vi "USBImageContinuousV1.4.vi"() -> ()   [LabVIEW 2019]
uses:
  C:/Users/Spenser Burrows/Desktop/Work/Labview software for spectrometer/PiezoStage_John/Piezojena.Protocols.Nv40Single.dll
  PiezoStage_John/Piezojena.Protocols.Nv40Single.dll
  <vilib>/Utility/file.llb/Write Delimited Spreadsheet (I64).vi
  Program Files (x86)/National Instruments/LabVIEW 2019/ATMCD32D.dll
  E:/PiezoStage_John/piezojena NV40Single.lvlib
panel:
  in  "Tab Control":T1(tab)
  out "Expected position on spectrometer (pixels):":dbl
  in  "Harmonic":dbl min=10.0 max=40.0
  out "l (nm)":dbl
  out "E (J)":dbl
  out "E (eV)":dbl
  out "Nearest Harmonic of 800nm":dbl
  out "Cursor Position (pixels)":dbl
  out "Distance to nearest harmonic of 800nm (pixels)":dbl
  in  "Grating:":u16(ring) items=["Shimadzu 30-006  "]
  in  "Laser:":u16(ring) items=["800nm  "]
  in  "Trigger":u32(ring) items=["Internal", "External"]
  out "Initialize":u32
  in  "Exposure Time (secs)":sgl format="%.2f"
  out "Calculated Exposure Value":sgl format="%.5f"
  out "Get Acquired Data":u32
  out "Start Acquisition":u32
  out "Detector X Pixels":i32
  out "Check Timings":u32
  out "Set Acquisition Mode":u32
  out "Set Readout Mode":u32
  out "Set Trigger Mode":u32
  out "Set Exposure Time":u32
  out "Get Detector":u32
  out "Detector Y Pixels":i32
  out "Shut Down":u32
  out "Set Gate Mode":u32
  out "Set Image":u32
  out "Raw Image From Camera":i32[][](graph)
  out "Vertical Binned Waveform Graph":i32[](graph)
  out "Get Status":u32
  in  "Stop":bool
  in  "Save image":bool
  out "Camera Status:":bool
  out "Last Image Saved:":string
  out "Wavelength Graph (nm)":cluster{"No prefix":dbl, i32}[](graph)
  out "Energy Graph (eV)":cluster{"eV":dbl, i32}[](graph)
  out "Harmonics Graph":cluster{"No prefix":dbl, i32}[](graph)
  in  "Measurement Length [fs]":ext=30.0
  out "Optical Cycles \nin measurement":ext=16.905589736842103296
  in  "Initial Piezo Position":sgl=40.0
  out "Number of Steps":ext=300.00000000000005795
  in  "Step Size [as]":sgl=100.0
  in  "?":bool
  in  "Settings":bool
  in  "Wavelength (nm)":i32(listbox)
  in  "Piezojena Seriel Port":refnum<visa-resource-name>="COM4"
  out "Piezo Voltage Supply":cluster{dbl[], dbl[]}(graph)={[0.0], [70.08999633789062]}
  in  "Initial Piezo Position [um]":dbl(slide)=40.0 scale=0.0..80.0
  in  "Final Piezo Position [um]":dbl(slide)=48.99377374 scale=0.0..80.0
  out "Volt Meter":dbl(knob)=70.08999633789062 scale=-10.0..150.0
  out "Raw Image From Camera":i32[][](graph)
  out "Status":u32
  # "Status"
  # "Return values"
  # "Acquisition Mode: Single Scan\nReadout Mode: Full Resolution Image"
  # "XUV Spectrometer Control VI"
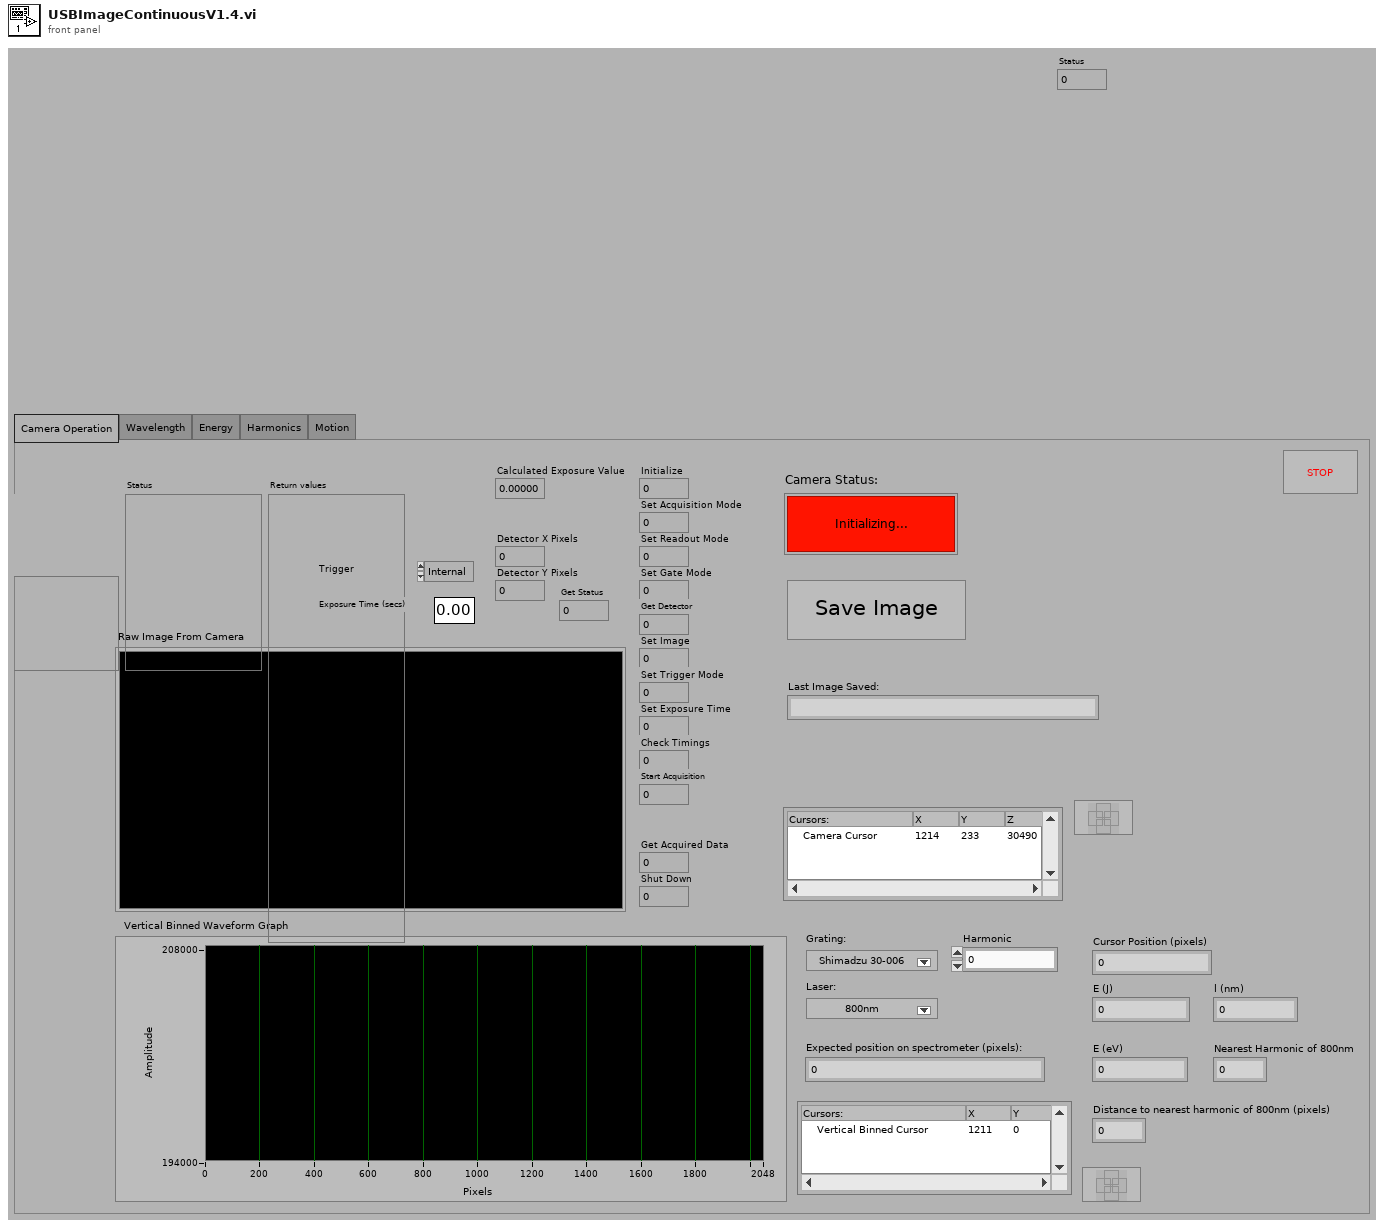
[diagram p1: front panel]
types:
  T1 = enum32{"Camera Operation", "Wavelength", "Energy", "Harmonics", "Motion"}
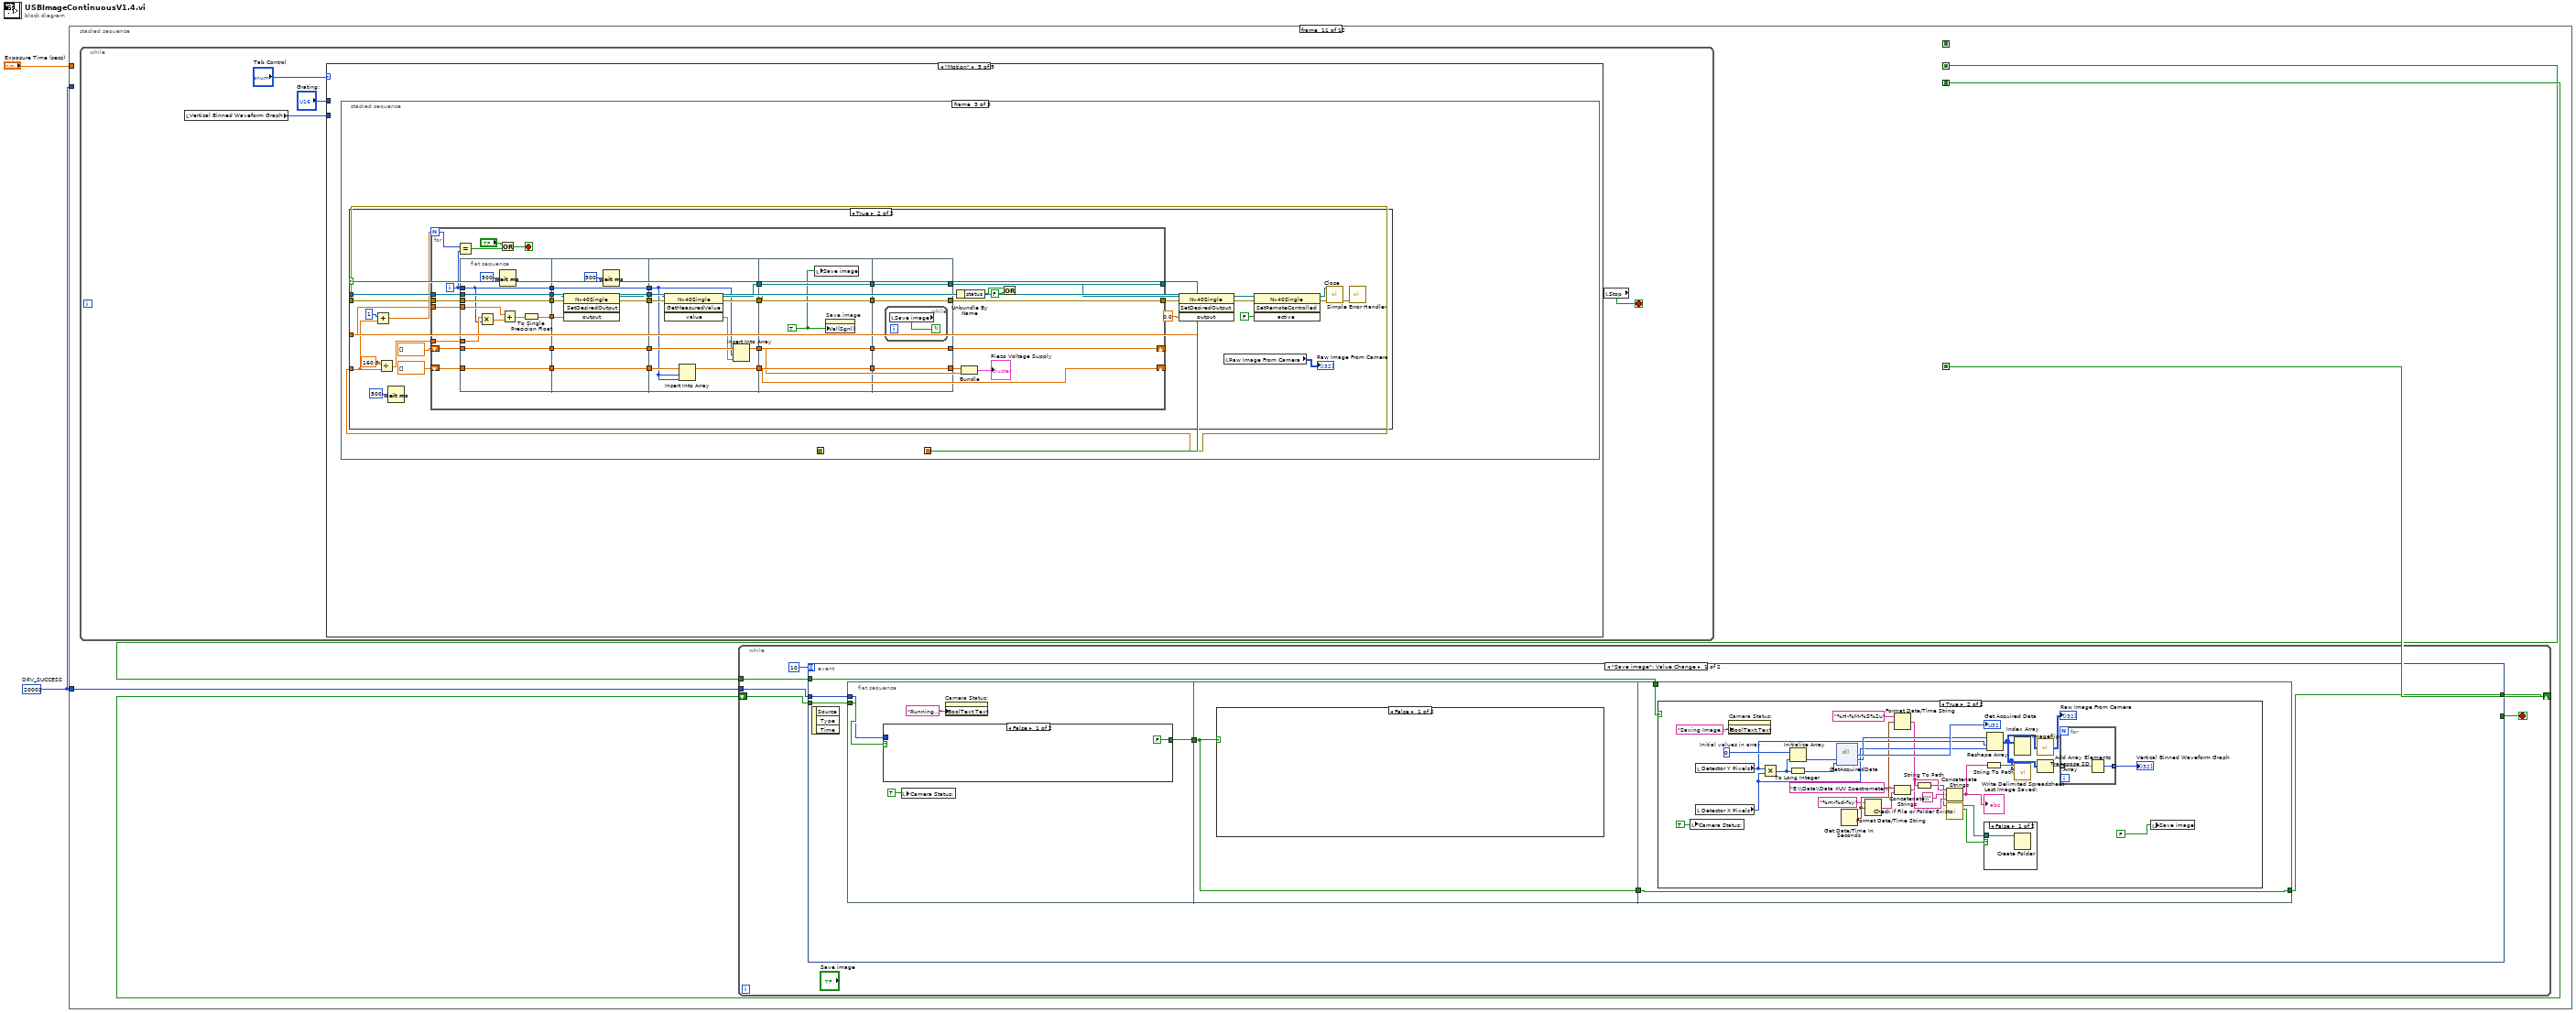
[diagram p0: block diagram]
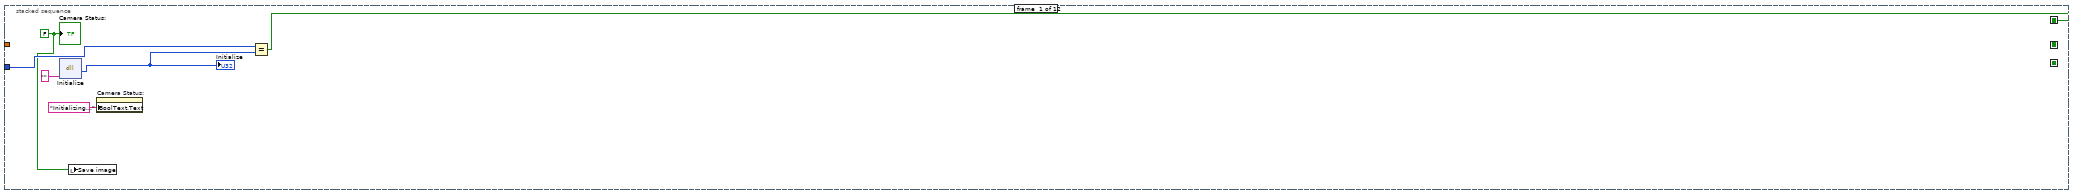
[diagram p2: hidden frame]
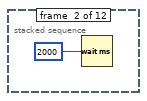
[diagram p3: hidden frame]
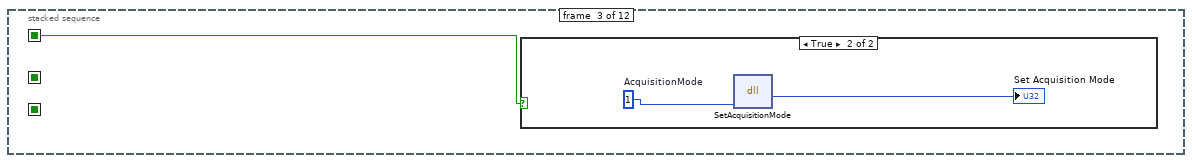
[diagram p4: hidden frame]
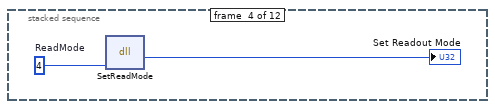
[diagram p6: hidden frame]
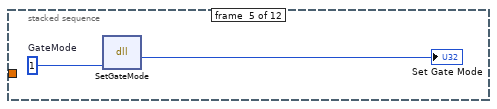
[diagram p7: hidden frame]
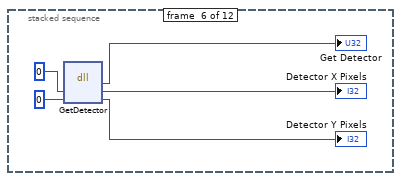
[diagram p8: hidden frame]
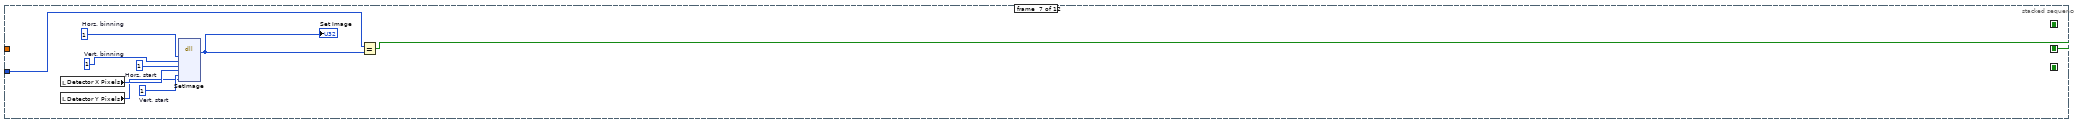
[diagram p9: hidden frame]
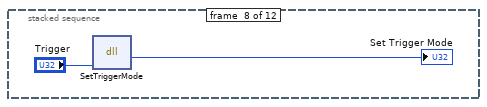
[diagram p10: hidden frame]
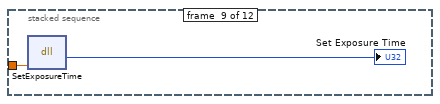
[diagram p11: hidden frame]
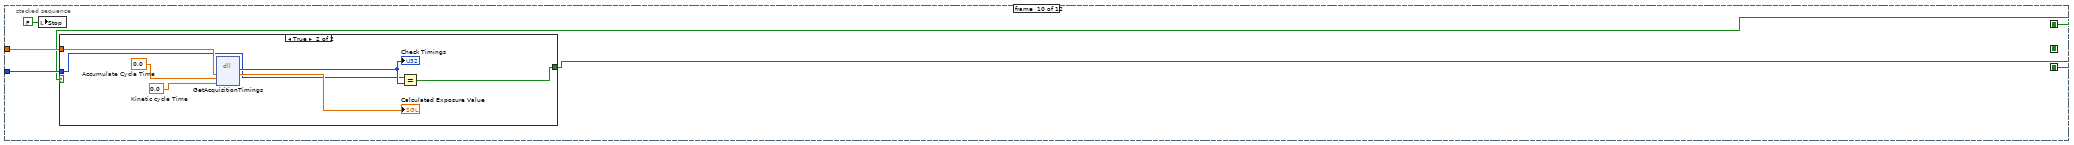
[diagram p12: hidden frame]
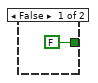
[diagram p13: hidden frame]
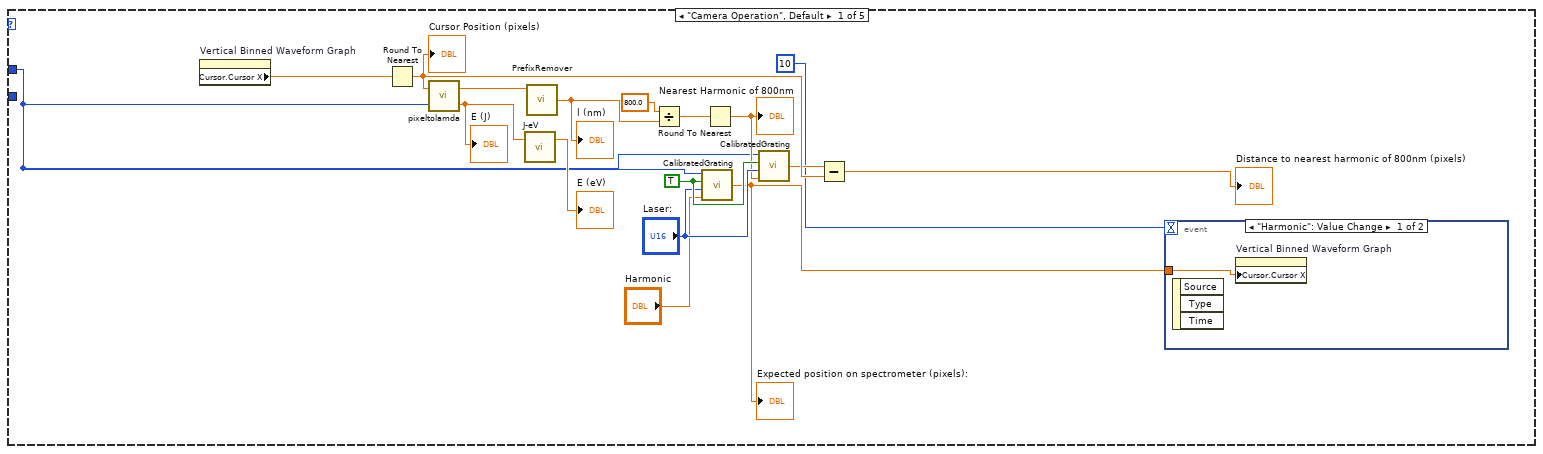
[diagram p14: hidden frame]
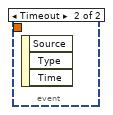
[diagram p15: hidden frame]
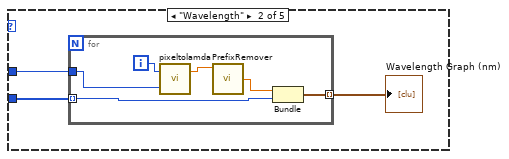
[diagram p16: hidden frame]
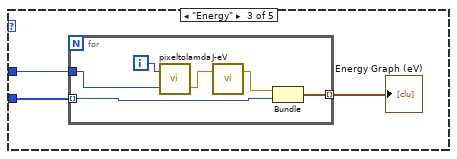
[diagram p17: hidden frame]
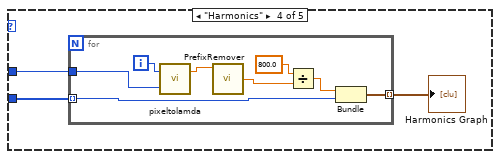
[diagram p18: hidden frame]
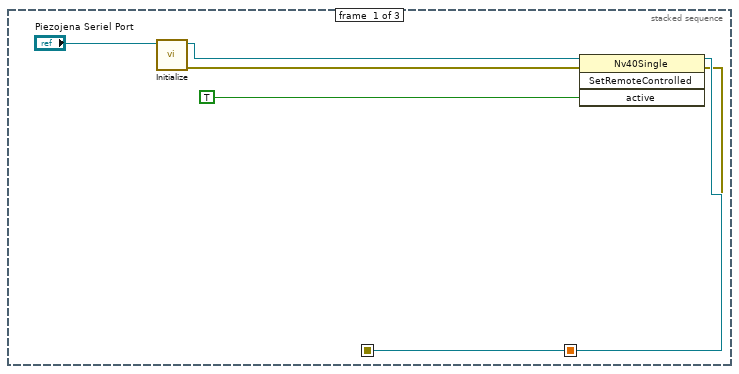
[diagram p19: hidden frame]
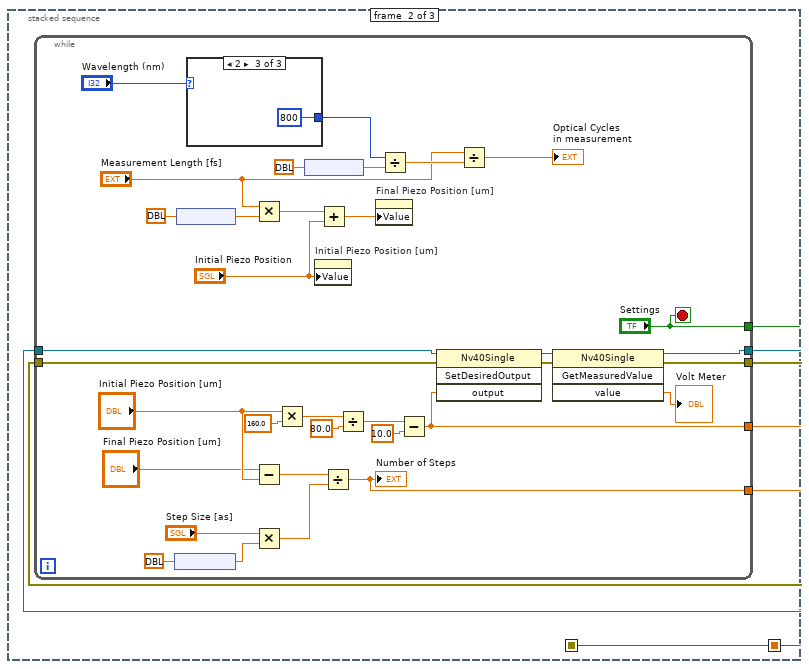
[diagram p20: hidden frame]
diagram:
  w1 = 20002  # DRV_SUCCESS
  n1 = stacked-sequence {
    seq-local: [w6 _ _ _ _ _ _ _ _ _ _ _] -> [_ _ w10 _ _ _ _ _ _ w36 _ w370]
    seq-local: [_ _ _ _ _ _ _ _ _ w37 _ _] -> [_ _ _ _ _ _ _ _ _ _ w51 _]
    seq-local: [_ _ _ _ _ _ _ _ _ _ w49 _] -> [_ _ _ _ _ _ _ _ _ _ _ _]
    seq-local: [_ _ _ _ _ _ w22 _ _ _ _ _] -> [_ _ _ _ _ _ _ _ _ _ w48 _]
    tunnel: "Exposure Time (secs)" -> [_ _ _ _ _ _ _ _ w34 w39 _ _]
    tunnel: w1 -> [w7 _ _ _ _ _ w24 _ _ w38 _ _]
    tunnel: w1 -> [_ _ _ _ _ _ _ _ _ _ w50 _]
    frame #0 {
      w3 = FALSE ("Camera Status:")
      n2 = dll-call lib="C:/Program Files (x86)/National Instruments/LabVIEW 2019/atmcd32d.dll" fn="Initialize" label="Call Library Function Initialize"("") -> (w8:u32)  [unwired: 4 in, 2 out]
      "Initialize" <- w8
      n3 = local write "Save image"(w3) -> ()
      n4 = property on="Camera Status:" class="Bool (strict)"("BoolText.Text"="Initializing..." ("String")) -> ()  [unwired: 2 in, 2 out]
      n5 = Equal?(x=w7, y=w8) -> (x = y?=w6:bool)
      "Camera Status:" <- w3
    }
    frame #1 {
      n6 = Wait (ms)(milliseconds to wait=u32 2000) -> ()  [unwired: 1 out]
    }
    frame #2 {
      n7 = case shown="True" w10 {
        frame False {
        }
        frame True {
          w12 = u16 1  # AcquisitionMode
          n8 = dll-call lib="C:/Program Files (x86)/National Instruments/LabVIEW 2019/atmcd32d.dll" fn="SetAcquisitionMode" label="Call Library Function SetAcquisitionMode"(w12) -> (→"Set Acquisition Mode":u32)  [unwired: 4 in, 2 out]
        }
      }
    }
    frame #3 {
      w14 = u16 4  # ReadMode
      n9 = dll-call lib="C:/Program Files (x86)/National Instruments/LabVIEW 2019/atmcd32d.dll" fn="SetReadMode" label="Call Library Function SetReadMode"(w14) -> (→"Set Readout Mode":u32)  [unwired: 4 in, 2 out]
    }
    frame #4 {
      w16 = u16 1  # GateMode
      n10 = dll-call lib="C:/Program Files (x86)/National Instruments/LabVIEW 2019/atmcd32d.dll" fn="SetGateMode" label="Call Library Function SetGateMode"(w16) -> (→"Set Gate Mode":u32)  [unwired: 4 in, 2 out]
    }
    frame #5 {
      n11 = dll-call lib="C:/Program Files (x86)/National Instruments/LabVIEW 2019/atmcd32d.dll" fn="GetDetector" label="Call Library FunctionGetDetector"(i16 0, i16 0) -> (→"Get Detector":u32, →"Detector X Pixels":i32, →"Detector Y Pixels":i32)  [unwired: 3 in, 2 out]
    }
    frame #6 {
      w27 = u16 1  # Vert. start
      w28 = u16 1  # Horz. start
      w29 = u16 1  # Vert. binning
      w30 = u16 1  # Horz. binning
      n12 = local read "Detector X Pixels"() -> (w26:i32)
      n13 = local read "Detector Y Pixels"() -> (w25:i32)
      n14 = dll-call lib="C:/Program Files (x86)/National Instruments/LabVIEW 2019/atmcd32d.dll" fn="SetImage" label="Call Library Function SetImage"(w30, w29, w28, w26, w27, w25) -> (w23:u32)  [unwired: 9 in, 2 out]
      "Set Image" <- w23
      n15 = Equal?(x=w24, y=w23) -> (x = y?=w22:bool)
    }
    frame #7 {
      n16 = dll-call lib="C:/Program Files (x86)/National Instruments/LabVIEW 2019/atmcd32d.dll" fn="SetTriggerMode" label="Call Library Function SetTrigger Mode"("Trigger") -> (→"Set Trigger Mode":u32)  [unwired: 4 in, 2 out]
    }
    frame #8 {
      n17 = dll-call lib="C:/Program Files (x86)/National Instruments/LabVIEW 2019/atmcd32d.dll" fn="SetExposureTime" label="Call Library FunctionSet Exposure Time"(w34) -> (→"Set Exposure Time":u32)  [unwired: 4 in, 2 out]
    }
    frame #9 {
      n18 = local write "Stop"(FALSE ("Stop")) -> ()
      n19 = case shown="True" w36 {
        tunnel: w39 -> [_ w44]
        tunnel: w38 -> [_ w41]
        tunnel: [FALSE w43] -> w37
        frame False {
        }
        frame True {
          w46 = sgl 0.0  # Accumulate Cycle Time
          w47 = sgl 0.0  # Kinetic cycle Time
          n20 = dll-call lib="C:/Program Files (x86)/National Instruments/LabVIEW 2019/atmcd32d.dll" fn="GetAcquisitionTimings" label="Call Library Function Check Timings"(w44, w46, w47) -> (w42:u32, →"Calculated Exposure Value":sgl)  [unwired: 5 in, 2 out]
          "Check Timings" <- w42
          n21 = Equal?(x=w41, y=w42) -> (x = y?=w43:bool)
        }
      }
    }
    frame #10 {
      n22 = while {
        stop <- w52 stop-if-true
        n23 = local read "Vertical Binned Waveform Graph"() -> (w54:i32[])
        n24 = case shown="\"Motion\"" "Tab Control" {
          tunnel: w54 -> [_ w76 w85 w94 _]
          tunnel: "Grating:" -> [w56 w75 w84 w93 _]
          frame "Camera Operation", Default {
            w72 = TRUE
            n25 = property on="Vertical Binned Waveform Graph" class="WFGraph (strict)"() -> ("Cursor.Cursor X"=w69:dbl)  [unwired: 2 in, 2 out]
            n26 = Round To Nearest(number=w69) -> (nearest integer value=w62:dbl)
            "Cursor Position (pixels)" <- w62
            n27 = call "pixeltolamda.vi"("Grating:"=w56, "Pixel Postion"=w62) -> ("E (J)"=w64:dbl, "lamda (m)"=w70:dbl)
            "E (J)" <- w64
            n28 = call "J-eV.vi"("J"=w64) -> ("eV"=→"E (eV)":dbl)  [unwired: 1 in, 1 out]
            n29 = call "PrefixRemover.vi"("Nano"=w70) -> ("No prefix"=w65:dbl)  [unwired: 3 in]
            "l (nm)" <- w65
            n30 = Divide(x=800.0, y=w65) -> (x/y=w67:dbl)
            n31 = call "CalibratedGrating.vi"("Harmonic"="Harmonic", "Laser:"="Laser:", "Subvi?"=w72, "Grating:"=w56) -> ("Position on spectrometer (pixels):"=w58:dbl)
            "Expected position on spectrometer (pixels):" <- w58
            n32 = Round To Nearest(number=w67) -> (nearest integer value=w61:dbl)
            "Nearest Harmonic of 800nm" <- w61
            n33 = call "CalibratedGrating.vi"("Harmonic"=w61, "Laser:"="Laser:", "Subvi?"=w72, "Grating:"=w56) -> ("Position on spectrometer (pixels):"=w60:dbl)
            n34 = Subtract(x=w60, y=w62) -> (x-y=→"Distance to nearest harmonic of 800nm (pixels)":dbl)
            n35 = event shown="[0] \"Harmonic\": Value Change" {
              selector: _ -> [_ _]
              dyn-events: _ -> [_ _]
              timeout: 10 -> [_ _]
              tunnel: w58 -> [w73 _]
              event "Harmonic": Value Change {
                n36 = event-data() -> ()  [unwired: 1 in, 3 out]
                n37 = property on="Vertical Binned Waveform Graph" class="WFGraph (strict)"("Cursor.Cursor X"=w73) -> ()  [unwired: 2 in, 2 out]
              }
              event Timeout {
                n38 = event-data() -> ()  [unwired: 1 in, 3 out]
              }
            }
          }
          frame "Wavelength" {
            n39 = for {
              tunnel: w76 -> [w78] mode=indexing
              tunnel: w75 -> [w80]
              tunnel: [w77] -> w74 mode=indexing
              i -> [w79]
              n40 = call "pixeltolamda.vi"("Grating:"=w80, "Pixel Postion"=w79) -> ("lamda (m)"=w81:dbl)  [unwired: 1 out]
              n41 = call "PrefixRemover.vi"("Nano"=w81) -> ("No prefix"=w82:dbl)  [unwired: 3 in]
              n42 = Bundle("No prefix"=w82, w78) -> (w77:cluster{"No prefix":dbl, i32})  [unwired: 1 in]
            }
            "Wavelength Graph (nm)" <- w74
          }
          frame "Energy" {
            n43 = for {
              tunnel: w85 -> [w87] mode=indexing
              tunnel: w84 -> [w90]
              tunnel: [w86] -> w83 mode=indexing
              i -> [w91]
              n44 = call "pixeltolamda.vi"("Grating:"=w90, "Pixel Postion"=w91) -> ("E (J)"=w89:dbl)  [unwired: 1 out]
              n45 = call "J-eV.vi"("J"=w89) -> ("eV"=w88:dbl)  [unwired: 1 in, 1 out]
              n46 = Bundle("eV"=w88, w87) -> (w86:cluster{"eV":dbl, i32})  [unwired: 1 in]
            }
            "Energy Graph (eV)" <- w83
          }
          frame "Harmonics" {
            n47 = for {
              tunnel: w94 -> [w99] mode=indexing
              tunnel: w93 -> [w101]
              tunnel: [w98] -> w92 mode=indexing
              i -> [w100]
              n48 = call "pixeltolamda.vi"("Grating:"=w101, "Pixel Postion"=w100) -> ("lamda (m)"=w102:dbl)  [unwired: 1 out]
              n49 = call "PrefixRemover.vi"("Nano"=w102) -> ("No prefix"=w96:dbl)  [unwired: 3 in]
              n50 = Divide(x=800.0, y=w96) -> (x/y=w95:dbl)
              n51 = Bundle(w95, w99) -> (w98:cluster{dbl, i32})  [unwired: 1 in]
            }
            "Harmonics Graph" <- w92
          }
          frame "Motion" {
            n52 = stacked-sequence {
              seq-local: [w104 _ _] -> [_ w115 _]
              seq-local: [w103 _ _] -> [_ w114 _]
              seq-local: [_ w113 _] -> [_ _ w157]
              seq-local: [_ w112 _] -> [_ _ w156]
              seq-local: [_ w111 _] -> [_ _ w155]
              seq-local: [_ w110 _] -> [_ _ w154]
              seq-local: [_ w109 _] -> [_ _ w153]
              frame #0 {
                n53 = call "Initialize.vi"("VISA resource name"="Piezojena Seriel Port") -> ("error out"=w108:errorcluster, "Piezojena.Protocols.Nv40Single.Nv40Single"=w107:refnum<k24>)  [unwired: 9 in]
                n54 = invoke class="Nv40Single" method="SetRemoteControlled"(reference=w107, error in=w108, "active"=TRUE) -> (reference out=w104:refnum<k24>, error out=w103:errorcluster)  [unwired: 1 in, 2 out]
              }
              frame #1 {
                n55 = while {
                  tunnel: ["Settings"] -> w113
                  tunnel: [w136] -> w112
                  tunnel: [w148] -> w111
                  tunnel: [w147] -> w110
                  tunnel: w115 -> [w146]
                  tunnel: w114 -> [w145]
                  tunnel: [w130] -> w109
                  stop <- "Settings" stop-if-true
                  n56 = node(ext[unit] 299792458.0) -> (w134:ext)
                  n57 = node(ext[unit] 299792458.0) -> (w121:ext)
                  n58 = case shown="2" "Wavelength (nm)" {
                    tunnel: [532 ("Numeric 2") 633 ("Numeric 2") 800 ("Numeric 2")] -> w125
                    frame 0, Default {
                    }
                    frame 1 {
                    }
                    frame 2 {
                    }
                  }
                  n59 = Multiply(x="Measurement Length [fs]", y=w121) -> (x*y=w119:ext)
                  n60 = Subtract(x="Final Piezo Position [um]", y="Initial Piezo Position [um]") -> (x-y=w133:dbl)
                  n61 = Multiply(x="Step Size [as]", y=w134) -> (x*y=w132:ext)
                  n62 = Multiply(x="Initial Piezo Position [um]", y=160.0 ("x")) -> (x*y=w139:dbl)
                  n63 = node(ext[unit] 299792458.0) -> (w124:ext)
                  n64 = property on="Initial Piezo Position [um]" class="Slide (strict)"("Value"="Initial Piezo Position") -> ()  [unwired: 2 in, 2 out]
                  n65 = Add(x=w119, y="Initial Piezo Position") -> (x+y=w118:ext)
                  n66 = Divide(x=w133, y=w132) -> (x/y=w130:ext)
                  "Number of Steps" <- w130
                  n67 = Divide(x=w139, y=80.0) -> (x/y=w138:dbl)
                  n68 = property on="Final Piezo Position [um]" class="Slide (strict)"("Value"=w118) -> ()  [unwired: 2 in, 2 out]
                  n69 = Divide(x=w125, y=w124) -> (x/y=w117:ext)
                  n70 = Subtract(x=w138, y=10.0) -> (x-y=w136:dbl)
                  n71 = invoke class="Nv40Single" method="SetDesiredOutput"(reference=w146, error in=w145, "output"=w136) -> (reference out=w142:refnum<k24>, error out=w143:errorcluster)  [unwired: 1 in, 2 out]
                  n72 = Divide(x="Measurement Length [fs]", y=w117) -> (x/y=→"Optical Cycles \nin measurement":ext)
                  n73 = invoke class="Nv40Single" method="GetMeasuredValue"(reference=w142, error in=w143) -> (reference out=w148:refnum<k24>, error out=w147:errorcluster, "value"=→"Volt Meter":sgl)  [unwired: 2 in, 1 out]
                }
              }
              frame #2 {
                n74 = case shown="True" w157 {
                  tunnel: w156 -> [_ w171]
                  tunnel: w155 -> [_ w170]
                  tunnel: w154 -> [_ w169]
                  tunnel: w153 -> [_ w165]
                  frame False {
                    (unwired) TRUE ("Stop Measurement 2")
                  }
                  frame True {
                    n75 = Add(x=1 ("y"), y=w165) -> (x+y=w172:ext)
                    n76 = Divide(x=160.0, y=w165) -> (x/y=w164:ext)
                    n77 = Wait (ms)(milliseconds to wait=u32 500 ("Wait for \nPiezo to start 2")) -> ()  [unwired: 1 out]
                    n78 = for {
                      N: w172 -> [w213]
                      tunnel: [w215] -> w163
                      tunnel: [w214] -> w162
                      tunnel: w170 -> [w205]
                      tunnel: w169 -> [w204]
                      tunnel: w171 -> [w200]
                      shift-right: [w188] -> _
                      shift-left: dbl[] [] -> [w198]
                      shift-right: [w189] -> _
                      shift-left: dbl[] [] -> [w193]
                      tunnel: w164 -> [w187]
                      i -> [w199]
                      stop <- w212 stop-if-true
                      n79 = Equal?(x=w213, y=w199) -> (x = y?=w211:bool)
                      n80 = flat-sequence {
                        tunnel: w204 -> [w225]
                        tunnel: w205 -> [w226]
                        tunnel: [w226] -> w203
                        tunnel: [w225] -> w202
                        tunnel: [w221] -> w201
                        tunnel: w199 -> [w218]
                        tunnel: w187 -> [w223]
                        tunnel: w200 -> [w222]
                        tunnel: w198 -> [w219]
                        tunnel: [w219] -> w197
                        tunnel: [w218] -> w194
                        tunnel: w193 -> [w216]
                        tunnel: [w216] -> w192
                        tunnel: [w231] -> w209
                        tunnel: [w230] -> w208
                        tunnel: w203 -> [w234]
                        tunnel: w202 -> [w233]
                        tunnel: w201 -> [w232]
                        tunnel: w197 -> [w229]
                        tunnel: [w229] -> w196
                        tunnel: [w228] -> w195
                        tunnel: w194 -> [w228]
                        tunnel: w192 -> [w227]
                        tunnel: [w227] -> w191
                        tunnel: w209 -> [w242]
                        tunnel: w208 -> [w241]
                        tunnel: w196 -> [w240]
                        tunnel: w195 -> [w237]
                        tunnel: w191 -> [w238]
                        tunnel: [w245] -> w186
                        tunnel: [w244] -> w185
                        tunnel: [w243] -> w184
                        tunnel: [w239] -> w183
                        tunnel: w186 -> [w250]
                        tunnel: w185 -> [w249]
                        tunnel: w184 -> [w248]
                        tunnel: w183 -> [w247]
                        tunnel: [w250] -> w182
                        tunnel: [w249] -> w181
                        tunnel: [w248] -> w180
                        tunnel: [w247] -> w179
                        tunnel: [w251] -> w189
                        tunnel: [w252] -> w188
                        tunnel: [w253] -> w214
                        tunnel: [w254] -> w215
                        tunnel: w182 -> [w254]
                        tunnel: w181 -> [w253]
                        tunnel: w180 -> [w252]
                        tunnel: w179 -> [w251]
                        frame #0 {
                          n81 = Multiply(x=w223, y=w218) -> (x*y=w217:ext)
                          n82 = Wait (ms)(milliseconds to wait=u32 500 ("Delay (ms) 3")) -> ()  [unwired: 1 out]
                          n83 = Add(x=w222, y=w217) -> (x+y=w224:ext)
                          n84 = To Single Precision Float(number=w224) -> (single precision float=w221:sgl)
                        }
                        frame #1 {
                          n85 = invoke class="Nv40Single" method="SetDesiredOutput"(reference=w234, error in=w233, "output"=w232) -> (reference out=w231:refnum<k24>, error out=w230:errorcluster)  [unwired: 1 in, 2 out]
                          n86 = Wait (ms)(milliseconds to wait=u32 500 ("Delay (ms) 4")) -> ()  [unwired: 1 out]
                        }
                        frame #2 {
                          n87 = invoke class="Nv40Single" method="GetMeasuredValue"(reference=w242, error in=w241) -> (reference out=w245:refnum<k24>, error out=w244:errorcluster, "value"=w236:sgl)  [unwired: 2 in, 1 out]
                          n88 = Insert Into Array(array=w238, index=w237, new element=w237) -> (w239:dbl[])
                          n89 = Insert Into Array(array=w240, index=w237, new element=w236) -> (w243:dbl[])
                        }
                        frame #3 {
                          w246 = TRUE
                          n90 = local write "Save image"(w246) -> ()
                          n91 = property on="Save image" class="Bool (strict)"("Val(Sgnl)"=w246) -> ()  [unwired: 2 in, 2 out]
                        }
                        frame #4 {
                          n92 = while {
                            stop <- w255 continue-if-true
                            n93 = local read "Save image"() -> (w255:bool)
                          }
                        }
                      }
                      n94 = Or(x="?", y=w211) -> (x .or. y?=w212:bool)
                      n95 = Unbundle By Name(w214) -> ("status"=w207:bool)
                      n96 = Bundle(w189, w188) -> (→"Piezo Voltage Supply":cluster{dbl[], dbl[]})  [unwired: 1 in]
                      n97 = Or(x=w207, y=FALSE ("Halt Measurment")) -> ()  [unwired: 1 out]
                    }
                    n98 = invoke class="Nv40Single" method="SetDesiredOutput"(reference=w163, error in=w162, "output"=sgl 0.0) -> (reference out=w160:refnum<k24>, error out=w159:errorcluster)  [unwired: 1 in, 2 out]
                    n99 = local read "Raw Image From Camera"() -> (→"Raw Image From Camera":i32[][])
                    n100 = invoke class="Nv40Single" method="SetRemoteControlled"(reference=w160, error in=w159, "active"=FALSE) -> (reference out=w177:refnum<k24>, error out=w175:errorcluster)  [unwired: 1 in, 2 out]
                    n101 = call "Close.vi"("error in (no error)"=w175, "reference"=w177) -> ("error out"=w178:errorcluster)  [unwired: 9 in]
                    n102 = call <vilib>:"Simple Error Handler.vi"("error in (no error)"=w178) -> ()  [unwired: 4 in, 5 out]
                  }
                }
              }
            }
          }
        }
        n103 = local read "Stop"() -> (w52:bool)
      }
      n104 = while {
        tunnel: w50 -> [w260]
        tunnel: w48 -> [w258]
        shift-right: [w259] -> w49
        shift-left: w51 -> [w261]
        stop <- w256 stop-if-true
        n105 = event shown="[0] \"Save image\": Value Change" {
          selector: _ -> [_ _]
          dyn-events: _ -> [_ _]
          timeout: 10 -> [_ _]
          tunnel: w261 -> [w265 w322]
          tunnel: w260 -> [w264 w321]
          tunnel: [w263 w320] -> w259
          tunnel: w258 -> [w262 w319]
          tunnel: [_ w318] -> w256
          event "Save image": Value Change {
            n106 = event-data() -> ()  [unwired: 1 in, 3 out]
            n107 = flat-sequence {
              tunnel: w265 -> [w272]
              tunnel: w264 -> [w271]
              tunnel: [w270] -> w267
              tunnel: w267 -> [w277]
              tunnel: [w277] -> w266
              tunnel: [w285] -> w263
              tunnel: w266 -> [w285]
              tunnel: w262 -> [w284]
              frame #0 {
                n108 = case shown="False" w272 {
                  tunnel: [FALSE w275] -> w270
                  tunnel: w271 -> [_ w274]
                  frame False {
                  }
                  frame True {
                    n109 = dll-call lib="C:/Program Files (x86)/National Instruments/LabVIEW 2019/atmcd32d.dll" fn="StartAcquisition" label="Call Library Function start acquisition"() -> (w276:u32)  [unwired: 3 in, 2 out]
                    "Start Acquisition" <- w276
                    n110 = Equal?(x=w274, y=w276) -> (x = y?=w275:bool)
                  }
                }
                n111 = local write "Camera Status:"(TRUE ("Camera Status:")) -> ()
                n112 = property on="Camera Status:" class="Bool (strict)"("BoolText.Text"="Running..." ("Boolean Text.Text")) -> ()  [unwired: 2 in, 2 out]
              }
              frame #1 {
                n113 = case shown="False" w277 {
                  frame False {
                  }
                  frame True {
                    n114 = while {
                      stop <- w281 continue-if-true
                      w280 = u16 20072  # DRV ACQUIRING
                      n115 = Wait Until Next ms Multiple(millisecond multiple=u32 500) -> ()  [unwired: 1 out]
                      n116 = dll-call lib="C:/Program Files (x86)/National Instruments/LabVIEW 2019/atmcd32d.dll" fn="GetStatus" label="Call Library Function GetAcquisitionStatus"(u16 0) -> (→"Get Status":u32, w279:u32)  [unwired: 3 in, 2 out]
                      "Status" <- w279
                      n117 = Equal?(x=w279, y=w280) -> (x = y?=w281:bool)
                    }
                  }
                }
              }
              frame #2 {
                n118 = case shown="True" w284 {
                  frame False {
                  }
                  frame True {
                    w313 = 0  # Initial values in array
                    n119 = local write "Camera Status:"(TRUE ("Camera Status:")) -> ()
                    n120 = local read "Detector Y Pixels"() -> (w307:i32)
                    n121 = local read "Detector X Pixels"() -> (w306:i32)
                    n122 = property on="Camera Status:" class="Bool (strict)"("BoolText.Text"="Saving Image..." ("Boolean Text.Text")) -> ()  [unwired: 2 in, 2 out]
                    n123 = Multiply(x=w307, y=w306) -> (x*y=w309:i32)
                    n124 = To Long Integer(number=w309) -> (32bit integer=w310:i32)
                    n125 = Initialize Array "Initialize Array"(w313, w309) -> (w311:i32[])
                    n126 = dll-call lib="C:/Program Files (x86)/National Instruments/LabVIEW 2019/atmcd32d.dll" fn="GetAcquiredData" label="Call Library Function Get Acquired data"(w311, w310) -> (→"Get Acquired Data":u32, w308:i32[])  [unwired: 4 in, 2 out]
                    n127 = Get Date/Time In Seconds() -> (seconds since 1Jan1904=w303:timestamp)
                    n128 = Format Date/Time String(time format string (%c)="%m-%d-%y", seconds (now)=w303) -> (date/time string=w301:string)  [unwired: 1 in]
                    n129 = Format Date/Time String(time format string (%c)="%H-%M-%S%2u", seconds (now)=w303) -> (date/time string=w302:string)  [unwired: 1 in]
                    n130 = Concatenate Strings("E:\\Data\\Data XUV Spectrometer\\" ("string"), w301) -> (w304:string)
                    n131 = String To Path(string=w304) -> (path=w300:path)
                    n132 = Concatenate Strings(w304, "\\" ("string"), w302) -> (w305:string)
                    "Last Image Saved:" <- w305
                    n133 = call <vilib>:"Check if File or Folder Exists.vi"("path"=w300) -> ("file or folder exists?"=w298:bool, "dup path"=w299:path)  [unwired: 8 in, 1 out]
                    n134 = case shown="False" w298 {
                      tunnel: w299 -> [w316 _]
                      frame False {
                        n135 = Create Folder(path (use dialog)=w316) -> ()  [unwired: 2 in, 3 out]
                      }
                      frame True {
                      }
                    }
                    n136 = String To Path(string=w305) -> (path=w293:path)
                    n137 = Reshape Array(w308, w307, w306) -> (w288:i32[][])
                    n138 = Index Array(array=w288) -> ()  [unwired: 2 in, 1 out]
                    n139 = call-poly <vilib>:"Write Delimited Spreadsheet.vi"("file path (dialog if empty)"=w293, "2D data"=w288) -> ()  [unwired: 12 in, 2 out]
                    n140 = call "Imageflip.vi"("2D array"=w288) -> ("transposed array"=→"Raw Image From Camera":i32[][])
                    n141 = Transpose 2D Array(2D array=w288) -> (transposed array=w292:i32[][])
                    n142 = for {
                      tunnel: w292 -> [w315] mode=indexing
                      tunnel: [w314] -> w291 mode=indexing
                      n143 = Add Array Elements(numeric array=w315) -> (sum=w314:i32)
                    }
                    "Vertical Binned Waveform Graph" <- w291
                    n144 = local write "Save image"(FALSE ("Take image")) -> ()
                  }
                }
              }
            }
          }
          event Timeout {
            n145 = event-data() -> ()  [unwired: 1 in, 3 out]
            n146 = flat-sequence {
              tunnel: w322 -> [w329]
              tunnel: w321 -> [w328]
              tunnel: [w327] -> w324
              tunnel: w324 -> [w334]
              tunnel: [w334] -> w323
              tunnel: w323 -> [w341]
              tunnel: w319 -> [w342]
              tunnel: [w341] -> w317
              tunnel: ["Stop"] -> w318
              tunnel: [w367] -> w320
              tunnel: w317 -> [w367]
              frame #0 {
                n147 = case shown="True" w329 {
                  tunnel: [FALSE w333] -> w327
                  tunnel: w328 -> [_ w332]
                  frame False {
                  }
                  frame True {
                    n148 = dll-call lib="C:/Program Files (x86)/National Instruments/LabVIEW 2019/atmcd32d.dll" fn="StartAcquisition" label="Call Library Function start acquisition"() -> (w331:u32)  [unwired: 3 in, 2 out]
                    n149 = local write "Start Acquisition"(w331) -> ()
                    n150 = Equal?(x=w332, y=w331) -> (x = y?=w333:bool)
                  }
                }
                n151 = local write "Camera Status:"(TRUE ("Camera Status:")) -> ()
                n152 = property on="Camera Status:" class="Bool (strict)"("BoolText.Text"="Running..." ("Boolean Text.Text")) -> ()  [unwired: 2 in, 2 out]
              }
              frame #1 {
                n153 = case shown="True" w334 {
                  frame False {
                  }
                  frame True {
                    n154 = while {
                      stop <- w338 continue-if-true
                      w337 = u16 20072  # DRV ACQUIRING
                      n155 = Wait Until Next ms Multiple(millisecond multiple=u32 500) -> ()  [unwired: 1 out]
                      n156 = dll-call lib="C:/Program Files (x86)/National Instruments/LabVIEW 2019/atmcd32d.dll" fn="GetStatus" label="Call Library Function GetAcquisitionStatus"(u16 0) -> (w336:u32, w335:u32)  [unwired: 3 in, 2 out]
                      n157 = local write "Status"(w335) -> ()
                      n158 = local write "Get Status"(w336) -> ()
                      n159 = Equal?(x=w335, y=w337) -> (x = y?=w338:bool)
                    }
                  }
                }
              }
              frame #2 {
                n160 = case shown="True" w342 {
                  frame False {
                  }
                  frame True {
                    w357 = 0  # Initial values in array
                    n161 = local read "Detector Y Pixels"() -> (w352:i32)
                    n162 = local read "Detector X Pixels"() -> (w351:i32)
                    n163 = Multiply(x=w352, y=w351) -> (x*y=w354:i32)
                    n164 = Initialize Array "Initialize Array"(w357, w354) -> (w356:i32[])
                    n165 = To Long Integer(number=w354) -> (32bit integer=w355:i32)
                    n166 = dll-call lib="C:/Program Files (x86)/National Instruments/LabVIEW 2019/atmcd32d.dll" fn="GetAcquiredData" label="Call Library Function Get Acquired data"(w356, w355) -> (w349:u32, w353:i32[])  [unwired: 4 in, 2 out]
                    n167 = local write "Get Acquired Data"(w349) -> ()
                    n168 = Reshape Array(w353, w352, w351) -> (w343:i32[][])
                    n169 = Index Array(array=w343) -> ()  [unwired: 2 in, 1 out]
                    n170 = Array Max & Min(array=w343) -> (max value=w347:i32)  [unwired: 3 out]
                    n171 = Transpose 2D Array(2D array=w343) -> (transposed array=w350:i32[][])
                    n172 = call "Imageflip.vi"("2D array"=w343) -> ("transposed array"=w344:i32[][])
                    n173 = local write "Raw Image From Camera"(w344) -> ()
                    n174 = for {
                      tunnel: w350 -> [w365] mode=indexing
                      tunnel: [w364] -> w348 mode=indexing
                      n175 = Add Array Elements(numeric array=w365) -> (sum=w364:i32)
                    }
                    n176 = Greater?(x=w347, y=64900) -> (0:w345:bool)
                    n177 = case shown="True" w345 {
                      frame False {
                      }
                      frame True {
                        n178 = local write "Camera Status:"(FALSE ("Camera Status:")) -> ()
                        n179 = property on="Camera Status:" class="Bool (strict)"("BoolText.Text"="Saturated!" ("Boolean Text.Text")) -> ()  [unwired: 2 in, 2 out]
                        n180 = Two Button Dialog(message="Camera is saturating! Reduce photon flux!", 1:"I've fixed it, and I want to continue" ("message"), 2:"Shut Down Camera" ("T button name (\"OK\")")) -> (T button?=w359:bool)
                        n181 = local write "Stop"(w359) -> ()
                      }
                    }
                    n182 = local write "Vertical Binned Waveform Graph"(w348) -> ()
                  }
                }
              }
              frame #3 {
              }
            }
          }
        }
      }
    }
    frame #11 {
      n183 = local write "Camera Status:"(FALSE ("Camera Status:")) -> ()
      n184 = property on="Camera Status:" class="Bool (strict)"("BoolText.Text"="Shutting Down..." ("Boolean Text.Text")) -> ()  [unwired: 2 in, 2 out]
      n185 = case shown="True" w370 {
        frame False {
        }
        frame True {
          n186 = dll-call lib="C:/Program Files (x86)/National Instruments/LabVIEW 2019/atmcd32d.dll" fn="ShutDown" label="Call Library Function Shutdown"() -> (→"Shut Down":u32)  [unwired: 3 in, 2 out]
        }
      }
    }
  }
